vi "GPS data to cluster.vi"(2 "Speed Threshold (km/h)":dbl, 3 "Gps raw data in":string) -> (0 "Arm System?":bool, 1 "GPS Cluster":cluster{"Lat":dbl, "Lon":dbl, "Speed":dbl})   [LabVIEW 2020]
uses:
  <vilib>/express/express arith-compare/Formula/XNode/ExpressFormulaBlockNode.xnode
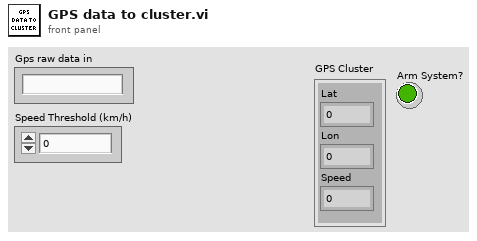
[diagram p1: front panel]
types:
  T1 = typedef "LVDateTimeRec.ctl" = cluster{"fractional second":dbl, "second":i32, "minute":i32, "hour":i32, "day of month":i32, "month":i32, "year":i32, "day of week":i32, "day of year":i32, "DST":i32}
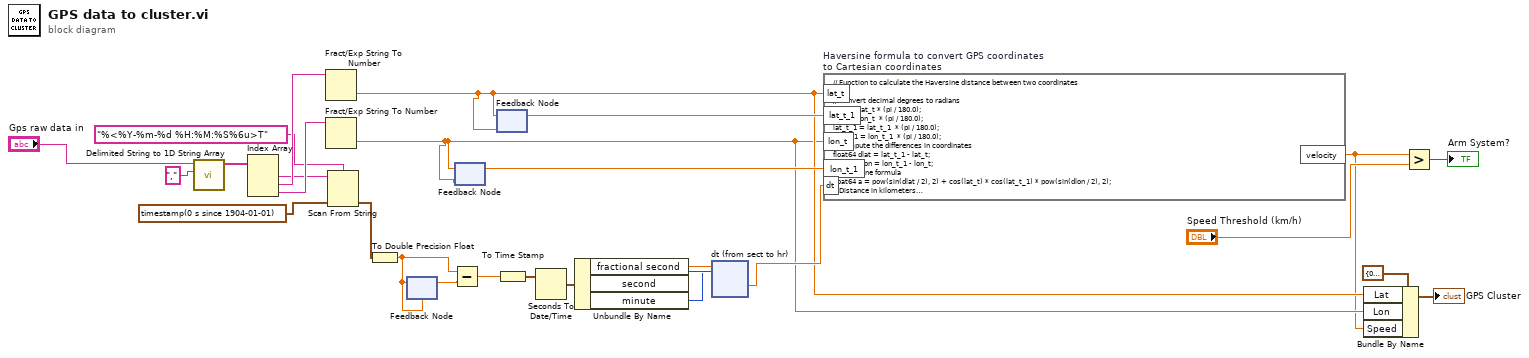
[diagram p0: block diagram]
diagram:
  n1 = call <vilib>:"Delimited String to 1D String Array.vi"("delimiter"=",", "delimited string"="Gps raw data in") -> ("string array"=w26:string[])  [unwired: 9 in]
  n2 = Index Array(array=w26) -> (element #1=w23:string, element #2=w24:string, element #3=w25:string)  [unwired: 3 in]
  n3 = Fract/Exp String To Number(string=w24) -> (number=w3:dbl)  [unwired: 3 in, 1 out]
  n4 = Fract/Exp String To Number(string=w25) -> (number=w2:dbl)  [unwired: 3 in, 1 out]
  n5 = Scan From String(format string="%<%Y-%m-%d %H:%M:%S%6u>T", input string=w23, default 1=timestamp(0 s since 1904-01-01) ("time stamp")) -> (output 1=w18:timestamp)  [unwired: 2 in, 3 out]
  n6 = To Double Precision Float(number=w18) -> (double precision float=w9:dbl)
  n7 = feedback #1(w9) -> (w8:dbl)
  n8 = feedback-in #1(w9) -> ()
  n9 = Subtract(x=w9, y=w8) -> (x-y=w19:dbl)
  n10 = feedback #2(w2) -> (w12:dbl)
  n11 = feedback-in #2(w2) -> ()
  n12 = feedback #3(w3) -> (w13:dbl)
  n13 = feedback-in #3(w3) -> ()
  n14 = To Time Stamp(1:w19) -> (0:w20:timestamp)
  n15 = Seconds To Date/Time(time stamp (now)=w20) -> (date time rec=w17:T1)  [unwired: 1 in]
  n16 = Unbundle By Name(w17) -> ("fractional second"=w16:dbl, "second"=w15:i32, "minute"=w14:i32)
  n17 = xnode "dt (from sect to hr)"("X1"=w16, "X2"=w15, "X3"=w14) -> ("Result"=w11:dbl)  [unwired: 1 in, 1 out]
  n18 = formula code="// Function to calculate the Haversine distance between two coordinates\n//\n// Convert decimal degrees to radians\nlat_t = lat_t * (pi / 180.0);\nlon_t =lon_t  * (pi / 180.0);\nlat_t_1 = lat_t_1  * (pi / 180.0);\nlon_t_1 = lon_t_1  * (pi / 180.0);\n// Compute the differences in coordinates\nfloat64 dlat = lat_t_1 - lat_t;\nfloat64 dlon = lon_t_1 - lon_t;\n// Haversine formula\nfloat64 a = pow(sin(dlat / 2), 2) + cos(lat_t) * cos(lat_t_1) * pow(sin(dlon / 2), 2);\n// Distance in kilometers\nfloat EARTH_RADIUS = 6371.0;\nfloat64 Cartesian_distance = EARTH_RADIUS * 2 * atan2(sqrt(a), sqrt(1- a));\nfloat64 velocity = Cartesian_distance / dt;" "Haversine formula to convert GPS coordinates to Cartesian coordinates"("lat_t"=w3, "lat_t_1"=w13, "lon_t"=w2, "lon_t_1"=w12, "dt"=w11) -> ("velocity"=w1:dbl)
  n19 = Bundle By Name(cluster=cluster{"Lat":dbl, "Lon":dbl, "Speed":dbl} {"Lat"=0.0, "Lon"=0.0, "Speed"=0.0} ("GPS"), "Lat"=w3, "Lon"=w2, "Speed"=w1) -> (→"GPS Cluster":cluster{"Lat":dbl, "Lon":dbl, "Speed":dbl})
  n20 = Greater?(x=w1, y="Speed Threshold (km/h)") -> (0:→"Arm System?":bool)
